vi "Frame.GetSignalRefs.vi"(8 "error in (no error)":errorcluster, 11 "Frame Item Ref in":T1 format="%.0x") -> (0 "error out":errorcluster, 1 "Child Refs":T1[](array[typedef]) format="%.0x", 2 "Signal Collection Ref out":T1=18446744073709551615 format="%.0x", 3 "Original Frame Ref out":T1 format="%.0x")   [LabVIEW 2019, in "Diagnostics Addon System Explorer.lvlib"]
uses:
  Diagnostics Addon System Explorer.lvlib
  <vilib>/NI VeriStand/Custom Device API/Custom Device Item Ref.ctl
  Shared/SubVIs/Constants.vi
  <vilib>/NI VeriStand/Custom Device Tools/Custom Device Utility Library/NI VeriStand - Search for Item by GUID.vi
  <vilib>/NI VeriStand/Custom Device API/Custom Device API.lvlib
  Shared/Diagnostics Addon Shared.lvlib
  <vilib>/NI VeriStand/Custom Device Tools/Custom Device Utility Library/Custom Device Utility Library.lvlib
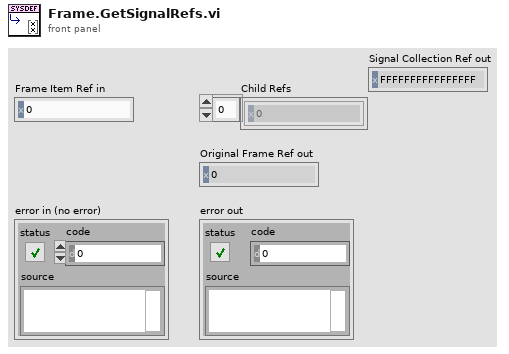
[diagram p1: front panel]
types:
  T1 = typedef "Custom Device API.lvlib/Custom Device Item Ref.ctl" = u64
  T2 = typedef "Custom Device API.lvlib/Custom Device Item Info.ctl" = cluster{"Name":string, "Is Channel":bool, "GUID":string, "Is Waveform":bool}
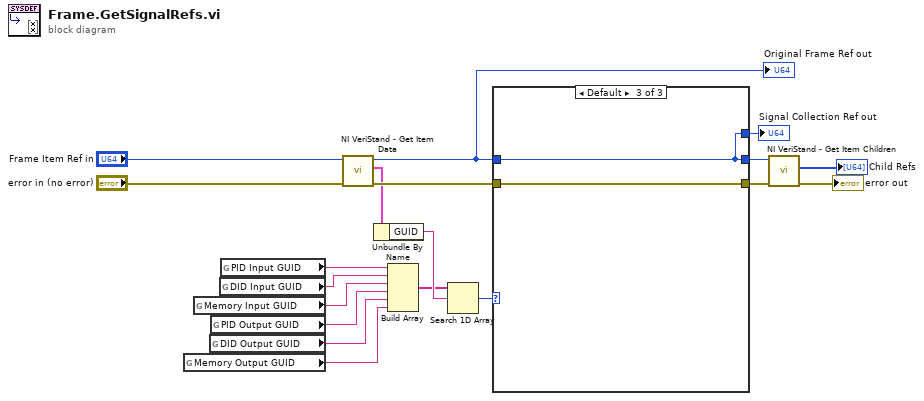
[diagram p0: block diagram]
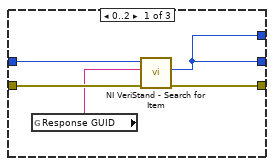
[diagram p2: hidden frame]
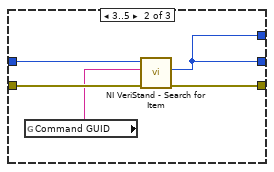
[diagram p3: hidden frame]
diagram:
  n1 = global read "Constants.vi" "Memory Output GUID"() -> (w12:string)
  n2 = global read "Constants.vi" "Memory Input GUID"() -> (w9:string)
  n3 = global read "Constants.vi" "DID Output GUID"() -> (w11:string)
  n4 = global read "Constants.vi" "PID Output GUID"() -> (w10:string)
  n5 = global read "Constants.vi" "DID Input GUID"() -> (w8:string)
  n6 = global read "Constants.vi" "PID Input GUID"() -> (w7:string)
  n7 = call <vilib>:"NI VeriStand - Get Item Data.vi"("error in (no error)"="error in (no error)", "Item Ref in"="Frame Item Ref in") -> ("error out"=w16:errorcluster, "Item Info"=w4:T2, "Item Ref out"=w19:T1)  [unwired: 7 out]
  "Original Frame Ref out" <- w19
  n8 = Unbundle By Name(w4) -> ("GUID"=w14:string)
  n9 = Build Array(w7, w8, w9, w10, w11, w12) -> (w13:string[])
  n10 = Search 1D Array(1D array=w13, element=w14) -> (index of element=w15:i32)  [unwired: 1 in]
  n11 = case shown="Default" w15 {
    tunnel: w16 -> [w24 w29 w31]
    tunnel: w19 -> [w23 w28 w30]
    tunnel: [w21 w27 w31] -> w17
    tunnel: [w20 w25 w30] -> w18
    tunnel: [w20 w25 w30] -> w1
    frame 0..2 {
      n12 = global read "Constants.vi" "Response GUID"() -> (w22:string)
      n13 = call-poly <vilib>:"NI VeriStand - Search for Item.vi"("error in"=w24, "Item GUID"=w22, "Section Ref in"=w23) -> ("error out"=w21:errorcluster, "Item Ref"=w20:T1)  [unwired: 5 in, 2 out]
    }
    frame 3..5 {
      n14 = global read "Constants.vi" "Command GUID"() -> (w26:string)
      n15 = call-poly <vilib>:"NI VeriStand - Search for Item.vi"("error in"=w29, "Item GUID"=w26, "Section Ref in"=w28) -> ("error out"=w27:errorcluster, "Item Ref"=w25:T1)  [unwired: 5 in, 2 out]
    }
    frame Default {
    }
  }
  "Signal Collection Ref out" <- w1
  n16 = call <vilib>:"NI VeriStand - Get Item Children.vi"("error in (no error)"=w17, "Item Ref in"=w18) -> ("error out"=→"error out":errorcluster, "Child Refs"=→"Child Refs":T1[])  [unwired: 6 in, 2 out]
